vi "Add VI or CTL to lvproj, lvlib, or lvclass.vi"(0 "Add into Project?":bool, 1 "VI Ref":refnum<vi>, 2 "lvlib or lvclass Ref":refnum<vi>, 5 "Add into lvlib or lvclass?":bool, 7 "Add into Virtual Folder?":bool, 9 "Virtual Folder Search Results":T3, 11 "error in":errorcluster, 12 "Initial State":T2, 13 "User VI Owner Status":T1, 14 "Project Name":string) -> (15 "error out":errorcluster)   [LabVIEW 2022 SP3]
doc: "This VI adds or inserts the newly created VI or CTL to a lvproj, lvlib, or lvclass, as per what the user selected. This VI can also insert the newly created VI or CTL into a Virtual Folder, if that's what the user selected.\n\nThis VI handles everything to do with inserting the newly created file into a Project Item.\n\nThis VI assumes that the newly created VI has already been saved to disk (i.e. already exists on disk).\n\nAcronyms\nATP = \"Add To Project?\" checkbox\nATO = \"Add To Owner?\" checkbox (lvlib or lvclass)\nATVF = \"Add To Virtual Folder?\" checkbox"
uses:
  DFS Output (cluster).ctl
  GUI Manager Module/Initial State (enum).ctl
  Owner Status (enum).ctl
  Virtual Folder Type (enum).ctl
panel:
  # "Development\ncontrols/indicators useful for development and testing, but which are not outputs of the VI"
  # "Input\nInputs to the VI"
  # "Output\nOutputs of the VI"
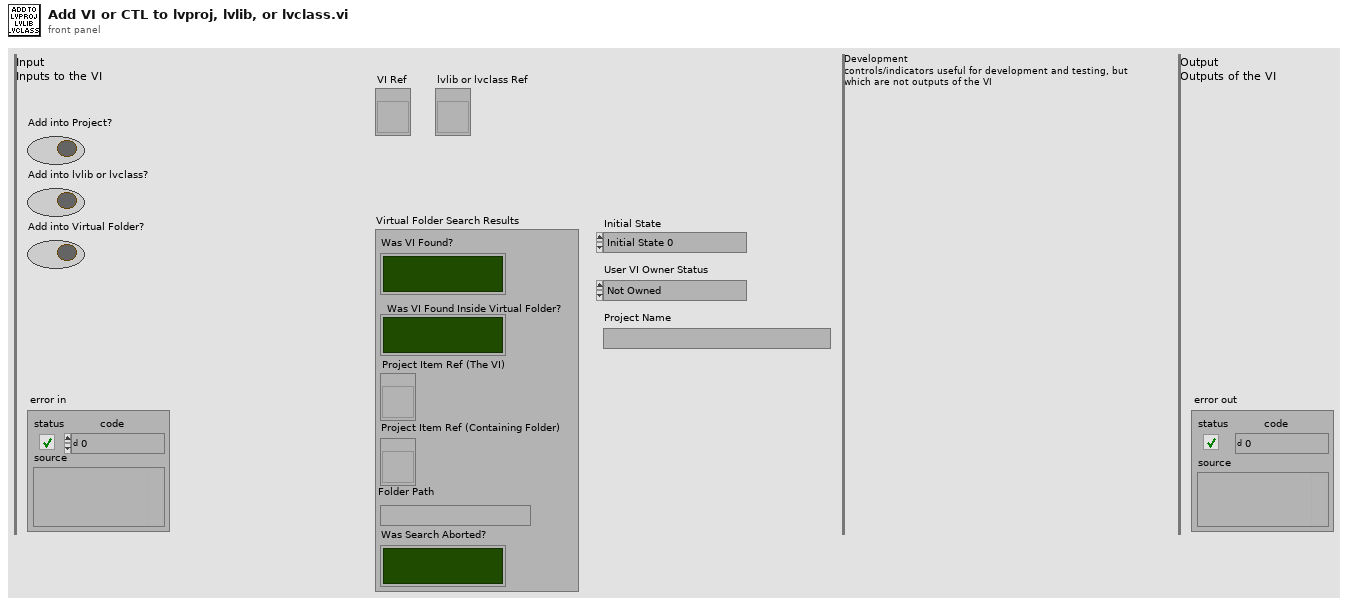
[diagram p1: front panel]
types:
  T1 = typedef "Owner Status (enum).ctl" = enum16{"Not Owned", "Owned by Library (lvlib)", "Owned by Class (lvclass)"}
  T2 = typedef "Initial State (enum).ctl" = enum16{"Initial State 0", "Initial State 1", "Initial State 2", "Initial State 3", "Initial State 4", "Initial State 5", "Initial State 6", "Initial State 7", "Initial State 8", "Initial State 9", "Initial State 10", "Initial State 11", "Initial State 12", "Initial State 13", "Initial State 14", "Initial State 15"}
  T3 = typedef "DFS Output (cluster).ctl" = cluster{"Was VI Found?":bool, "Was VI Found Inside Virtual Folder?":bool, "Project Item Ref (The VI)":refnum<vi>, "Project Item Ref (Containing Folder)":refnum<vi>, "Folder Path":string, "Was Search Aborted?":bool}
  T4 = typedef "Virtual Folder Type (enum).ctl" = enum16{"Owned by lvlib or lvclass", "Owned by lvproj"}
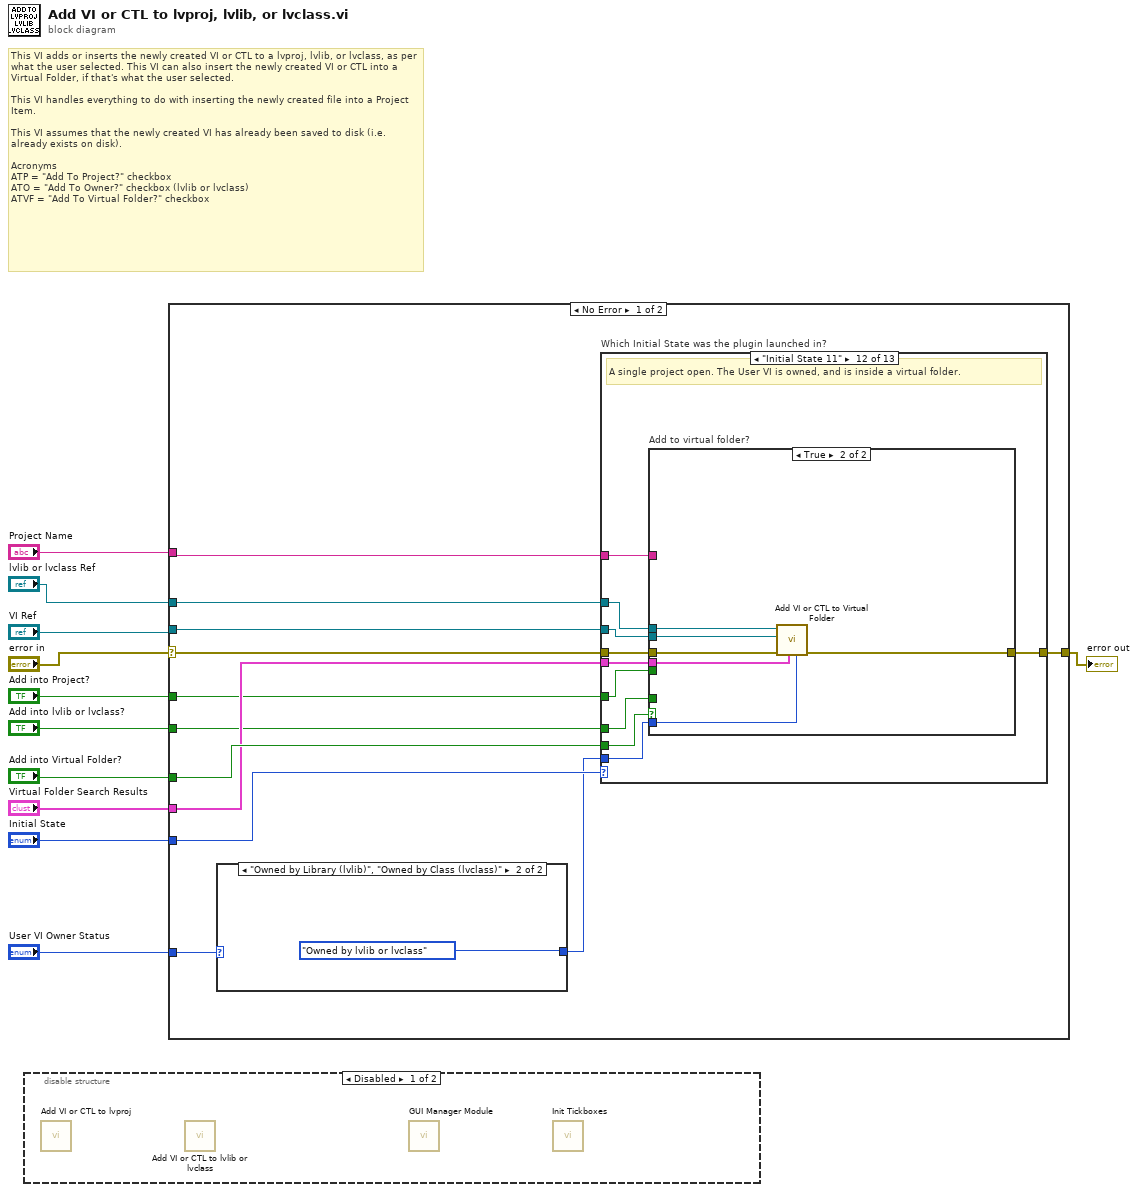
[diagram p0: block diagram]
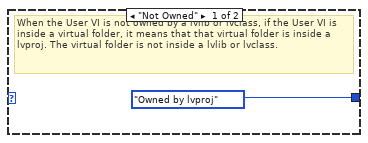
[diagram p2: hidden frame]
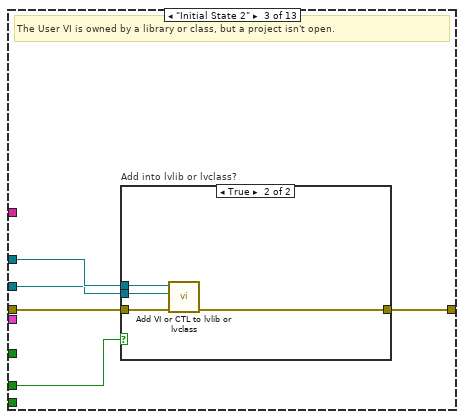
[diagram p5: hidden frame]
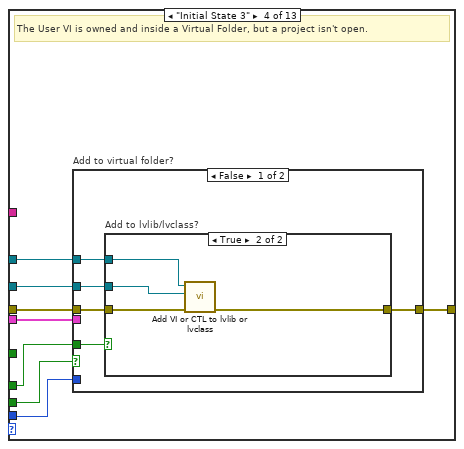
[diagram p7: hidden frame]
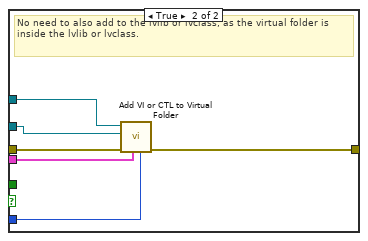
[diagram p9: hidden frame]
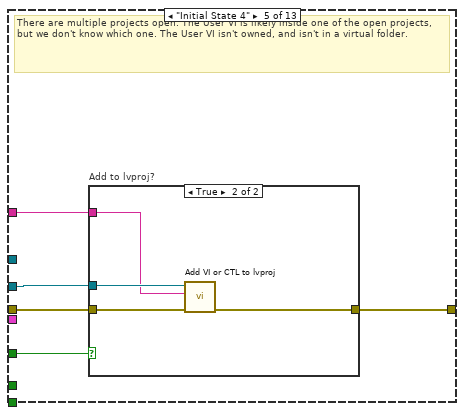
[diagram p10: hidden frame]
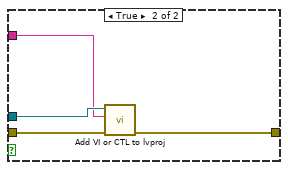
[diagram p14: hidden frame]
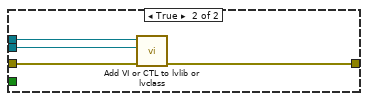
[diagram p15: hidden frame]
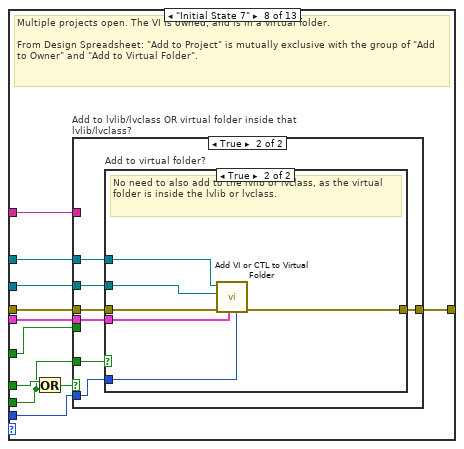
[diagram p16: hidden frame]
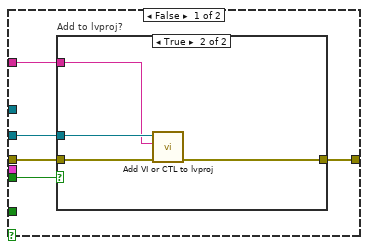
[diagram p17: hidden frame]
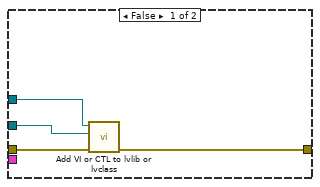
[diagram p19: hidden frame]
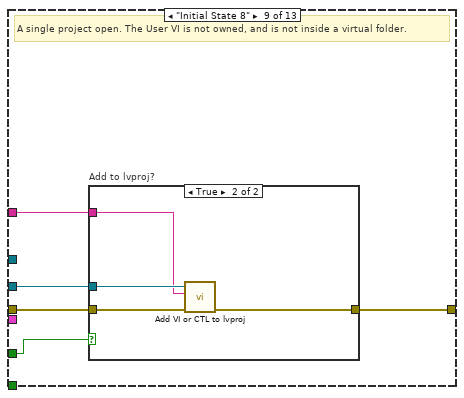
[diagram p20: hidden frame]
diagram:
  # "This VI adds or inserts the newly created VI or CTL to a lvproj, lvlib, or lvclass, as per what the user selected. This VI can also insert the newly created VI or CTL into a Virtual Folder, if that's what the user selected.\n\nThis VI handles everything to do with inserting the newly created file into a Project Item.\n\nThis VI assumes that the newly created VI has already been saved to disk (i.e. already exists on disk).\n\nAcronyms\nATP = \"Add To Project?\" checkbox\nATO = \"Add To Owner?\" checkbox (lvlib or lvclass)\nATVF = \"Add To Virtual Folder?\" checkbox"
  n1 = disable-structure shown="Disabled" {
    frame Disabled {
      n2 = call "Add VI or CTL to lvproj.vi"() -> ()  [unwired: 11 in, 1 out]
      n3 = call "Add VI or CTL to lvlib or lvclass.vi"() -> ()  [unwired: 11 in, 1 out]
      n4 = call "GUI Manager Module.vi"() -> ()  [unwired: 11 in, 1 out]
      n5 = call "Init Tickboxes.vi"() -> ()  [unwired: 11 in, 1 out]
    }
    frame Enabled {
    }
  }
  n6 = case shown="No Error" "error in" {
    selector: "error in" -> [w23 w226]
    tunnel: [w21 w226] -> w10
    tunnel: "lvlib or lvclass Ref" -> [w20 _]
    tunnel: "VI Ref" -> [w19 _]
    tunnel: "Virtual Folder Search Results" -> [w17 _]
    tunnel: "Add into Virtual Folder?" -> [w18 _]
    tunnel: "Initial State" -> [w22 _]
    tunnel: "Add into Project?" -> [w13 _]
    tunnel: "Add into lvlib or lvclass?" -> [w16 _]
    tunnel: "User VI Owner Status" -> [w15 _]
    tunnel: "Project Name" -> [w12 _]
    frame No Error {
      n7 = case shown="\"Owned by Library (lvlib)\", \"Owned by Class (lvclass)\"" w15 {
        tunnel: [Virtual_Folder_Type_(enum)."Owned by lvproj" ("Virtual Folder Type") Virtual_Folder_Type_(enum)."Owned by lvlib or lvclass" ("Virtual Folder Type")] -> w14
        frame "Not Owned" {
          # "When the User VI is not owned by a lvlib or lvclass, if the User VI is inside a virtual folder, it means that that virtual folder is inside a lvproj. The virtual folder is not inside a lvlib or lvclass."
        }
        frame "Owned by Library (lvlib)", "Owned by Class (lvclass)" {
        }
      }
      n8 = case "Which Initial State was the plugin launched in?" shown="\"Initial State 11\"" w22 {
        tunnel: w23 -> [w26 w27 w31 w45 w66 w72 w79 w104 w136 w150 w173 w197 w225]
        tunnel: [w26 w27 w32 w44 w65 w72 w78 w103 w135 w149 w172 w196 w225] -> w21
        tunnel: w20 -> [_ _ w30 w39 _ _ w77 w94 _ w144 w170 w195 _]
        tunnel: w19 -> [_ _ w29 w38 w63 _ w76 w98 w133 w145 w169 w194 _]
        tunnel: w18 -> [_ _ _ w43 _ _ _ w97 _ w148 _ w192 _]
        tunnel: w17 -> [_ _ _ w41 _ _ _ w96 _ w143 _ w191 _]
        tunnel: w16 -> [_ _ w28 w40 _ _ w75 w102 _ _ w171 w188 _]
        tunnel: w14 -> [_ _ _ w42 _ _ _ w95 _ w142 _ w190 _]
        tunnel: w13 -> [_ _ _ _ w64 _ w74 w100 w134 w147 w167 w189 _]
        tunnel: w12 -> [_ _ _ _ w62 _ w73 w99 w132 w146 w168 w193 _]
        frame "Initial State 0" {
          # "Do nothing. The ATP, ATO, and ATVF checkboxes should be disabled."
          # "The User VI is opened on its own. It's not part of a library, class, or project."
        }
        frame "Initial State 1" {
          # "Impossible Initial State. Expected to never occur."
        }
        frame "Initial State 2" {
          # "The User VI is owned by a library or class, but a project isn't open."
          n9 = case "Add into lvlib or lvclass?" shown="True" w28 {
            tunnel: [w33 w37] -> w32
            tunnel: w31 -> [w33 w36]
            tunnel: w30 -> [_ w35]
            tunnel: w29 -> [_ w34]
            frame False {
            }
            frame True {
              n10 = call "Add VI or CTL to lvlib or lvclass.vi"("error in"=w36, "VI Ref"=w34, "lvlib or lvclass Ref"=w35) -> ("error out"=w37:errorcluster)  [unwired: 8 in]
            }
          }
        }
        frame "Initial State 3" {
          # "The User VI is owned and inside a Virtual Folder, but a project isn't open."
          n11 = case "Add to virtual folder?" shown="False" w43 {
            tunnel: w45 -> [w50 w61]
            tunnel: [w49 w60] -> w44
            tunnel: w42 -> [_ w59]
            tunnel: w41 -> [_ w58]
            tunnel: w40 -> [w48 _]
            tunnel: w39 -> [w47 w57]
            tunnel: w38 -> [w46 w56]
            frame False {
              n12 = case "Add to lvlib/lvclass?" shown="True" w48 {
                tunnel: w50 -> [w51 w55]
                tunnel: [w51 w54] -> w49
                tunnel: w47 -> [_ w53]
                tunnel: w46 -> [_ w52]
                frame False {
                  # "The user selected not to insert the newly created VI anywhere."
                }
                frame True {
                  n13 = call "Add VI or CTL to lvlib or lvclass.vi"("error in"=w55, "VI Ref"=w52, "lvlib or lvclass Ref"=w53) -> ("error out"=w54:errorcluster)  [unwired: 8 in]
                }
              }
            }
            frame True {
              # "No need to also add to the lvlib or lvclass, as the virtual folder is inside the lvlib or lvclass."
              n14 = call "Add VI or CTL to Virtual Folder.vi"("Virtual Folder Type"=w59, "Virtual Folder Search Results"=w58, "error in"=w61, "VI Ref"=w56, "lvlib or lvclass Ref"=w57) -> ("error out"=w60:errorcluster)  [unwired: 6 in]
            }
          }
        }
        frame "Initial State 4" {
          # "There are multiple projects open. The User VI is likely inside one of the open projects, but we don't know which one. The User VI isn't owned, and isn't in a virtual folder."
          n15 = case "Add to lvproj?" shown="True" w64 {
            tunnel: w66 -> [w67 w71]
            tunnel: [w67 w70] -> w65
            tunnel: w63 -> [_ w69]
            tunnel: w62 -> [_ w68]
            frame False {
              # "The user selected not to insert the newly created VI anywhere."
            }
            frame True {
              n16 = call "Add VI or CTL to lvproj.vi"("error in"=w71, "Project Name"=w68, "Reference of newly created VI or CTL"=w69) -> ("error out"=w70:errorcluster)  [unwired: 8 in]
            }
          }
        }
        frame "Initial State 5" {
          # "Impossible Initial State. Expected to never occur."
        }
        frame "Initial State 6" {
          # "Multiple projects open. The VI is owned, but isn't in a virtual folder.\n\nFrom Design Spreadsheet: Ticking \"Add to Owner\" and \"Add to Project\" is mutually exclusive (only one checkbox can be ticked at a given time)"
          n17 = case "Add to lvlib/lvclass?" shown="False" w75 {
            tunnel: w79 -> [w84 w93]
            tunnel: [w83 w92] -> w78
            tunnel: w77 -> [_ w91]
            tunnel: w76 -> [w81 w90]
            tunnel: w74 -> [w82 _]
            tunnel: w73 -> [w80 _]
            frame False {
              n18 = case "Add to lvproj?" shown="False" w82 {
                tunnel: w84 -> [w85 w89]
                tunnel: [w85 w88] -> w83
                tunnel: w81 -> [_ w87]
                tunnel: w80 -> [_ w86]
                frame False {
                  # "The user selected not to insert the newly created VI anywhere."
                }
                frame True {
                  n19 = call "Add VI or CTL to lvproj.vi"("error in"=w89, "Project Name"=w86, "Reference of newly created VI or CTL"=w87) -> ("error out"=w88:errorcluster)  [unwired: 8 in]
                }
              }
            }
            frame True {
              n20 = call "Add VI or CTL to lvlib or lvclass.vi"("error in"=w93, "VI Ref"=w90, "lvlib or lvclass Ref"=w91) -> ("error out"=w92:errorcluster)  [unwired: 8 in]
            }
          }
        }
        frame "Initial State 7" {
          # "Multiple projects open. The VI is owned, and is in a virtual folder.\n\nFrom Design Spreadsheet: \"Add to Project\" is mutually exclusive with the group of \"Add to Owner\" and \"Add to Virtual Folder\"."
          n21 = Or(x=w102, y=w97) -> (x .or. y?=w101:bool)
          n22 = case "Add to lvlib/lvclass OR virtual folder inside that lvlib/lvclass?" shown="True" w101 {
            tunnel: [w108 w120] -> w103
            tunnel: w104 -> [w109 w121]
            tunnel: w100 -> [w107 _]
            tunnel: w99 -> [w106 _]
            tunnel: w98 -> [w105 w116]
            tunnel: w97 -> [_ w119]
            tunnel: w96 -> [_ w118]
            tunnel: w95 -> [_ w117]
            tunnel: w94 -> [_ w115]
            frame False {
              n23 = case "Add to lvproj?" shown="True" w107 {
                tunnel: w109 -> [w110 w114]
                tunnel: [w110 w113] -> w108
                tunnel: w105 -> [_ w112]
                tunnel: w106 -> [_ w111]
                frame False {
                  # "The user selected not to insert the newly created VI anywhere."
                }
                frame True {
                  n24 = call "Add VI or CTL to lvproj.vi"("error in"=w114, "Project Name"=w111, "Reference of newly created VI or CTL"=w112) -> ("error out"=w113:errorcluster)  [unwired: 8 in]
                }
              }
            }
            frame True {
              n25 = case "Add to virtual folder?" shown="True" w119 {
                tunnel: w121 -> [w125 w131]
                tunnel: [w124 w130] -> w120
                tunnel: w117 -> [_ w129]
                tunnel: w118 -> [_ w128]
                tunnel: w115 -> [w123 w126]
                tunnel: w116 -> [w122 w127]
                frame False {
                  n26 = call "Add VI or CTL to lvlib or lvclass.vi"("error in"=w125, "VI Ref"=w122, "lvlib or lvclass Ref"=w123) -> ("error out"=w124:errorcluster)  [unwired: 8 in]
                }
                frame True {
                  # "No need to also add to the lvlib or lvclass, as the virtual folder is inside the lvlib or lvclass."
                  n27 = call "Add VI or CTL to Virtual Folder.vi"("Virtual Folder Type"=w129, "Virtual Folder Search Results"=w128, "error in"=w131, "VI Ref"=w127, "lvlib or lvclass Ref"=w126) -> ("error out"=w130:errorcluster)  [unwired: 6 in]
                }
              }
            }
          }
        }
        frame "Initial State 8" {
          # "A single project open. The User VI is not owned, and is not inside a virtual folder."
          n28 = case "Add to lvproj?" shown="True" w134 {
            tunnel: w136 -> [w137 w141]
            tunnel: [w137 w140] -> w135
            tunnel: w133 -> [_ w139]
            tunnel: w132 -> [_ w138]
            frame False {
              # "The user selected not to insert the newly created VI anywhere."
            }
            frame True {
              n29 = call "Add VI or CTL to lvproj.vi"("error in"=w141, "Project Name"=w138, "Reference of newly created VI or CTL"=w139) -> ("error out"=w140:errorcluster)  [unwired: 8 in]
            }
          }
        }
        frame "Initial State 9" {
          # "A single project open. The User VI is not owned, but is inside a virtual folder."
          n30 = case "Add to virtual folder?" shown="False" w148 {
            tunnel: w150 -> [w155 w166]
            tunnel: [w154 w165] -> w149
            tunnel: w144 -> [_ w164]
            tunnel: w145 -> [w152 w163]
            tunnel: w147 -> [w153 _]
            tunnel: w146 -> [w151 _]
            tunnel: w143 -> [_ w162]
            tunnel: w142 -> [_ w161]
            frame False {
              n31 = case "Add to lvproj?" shown="True" w153 {
                tunnel: w155 -> [w156 w160]
                tunnel: [w156 w159] -> w154
                tunnel: w152 -> [_ w158]
                tunnel: w151 -> [_ w157]
                frame False {
                  # "The user selected not to insert the newly created VI anywhere."
                }
                frame True {
                  n32 = call "Add VI or CTL to lvproj.vi"("error in"=w160, "Project Name"=w157, "Reference of newly created VI or CTL"=w158) -> ("error out"=w159:errorcluster)  [unwired: 8 in]
                }
              }
            }
            frame True {
              n33 = call "Add VI or CTL to Virtual Folder.vi"("Virtual Folder Type"=w161, "Virtual Folder Search Results"=w162, "error in"=w166, "VI Ref"=w163, "lvlib or lvclass Ref"=w164) -> ("error out"=w165:errorcluster)  [unwired: 6 in]
            }
          }
        }
        frame "Initial State 10" {
          # "A single project open. The User VI is owned, but is not inside a virtual folder."
          n34 = case "Add to lvlib/lvclass?" shown="False" w171 {
            tunnel: w173 -> [w178 w187]
            tunnel: [w177 w186] -> w172
            tunnel: w170 -> [_ w185]
            tunnel: w169 -> [w175 w184]
            tunnel: w167 -> [w176 _]
            tunnel: w168 -> [w174 _]
            frame False {
              n35 = case "Add to lvproj?" shown="False" w176 {
                tunnel: w178 -> [w179 w183]
                tunnel: [w179 w182] -> w177
                tunnel: w175 -> [_ w181]
                tunnel: w174 -> [_ w180]
                frame False {
                  # "The user selected not to insert the newly created VI anywhere."
                }
                frame True {
                  n36 = call "Add VI or CTL to lvproj.vi"("error in"=w183, "Project Name"=w180, "Reference of newly created VI or CTL"=w181) -> ("error out"=w182:errorcluster)  [unwired: 8 in]
                }
              }
            }
            frame True {
              n37 = call "Add VI or CTL to lvlib or lvclass.vi"("error in"=w187, "VI Ref"=w184, "lvlib or lvclass Ref"=w185) -> ("error out"=w186:errorcluster)  [unwired: 8 in]
            }
          }
        }
        frame "Initial State 11" {
          # "A single project open. The User VI is owned, and is inside a virtual folder."
          n38 = case "Add to virtual folder?" shown="True" w192 {
            tunnel: w197 -> [w204 w224]
            tunnel: [w203 w223] -> w196
            tunnel: w195 -> [w198 w222]
            tunnel: w194 -> [w201 w221]
            tunnel: w189 -> [w202 _]
            tunnel: w193 -> [w200 _]
            tunnel: w191 -> [_ w220]
            tunnel: w190 -> [_ w219]
            tunnel: w188 -> [w199 _]
            frame False {
              n39 = case "Add to lvlib/lvclass?" shown="False" w199 {
                tunnel: w204 -> [w209 w218]
                tunnel: [w208 w217] -> w203
                tunnel: w202 -> [w207 _]
                tunnel: w201 -> [w206 w215]
                tunnel: w200 -> [w205 _]
                tunnel: w198 -> [_ w216]
                frame False {
                  n40 = case "Add to lvproj?" shown="False" w207 {
                    tunnel: w209 -> [w210 w214]
                    tunnel: [w210 w213] -> w208
                    tunnel: w206 -> [_ w212]
                    tunnel: w205 -> [_ w211]
                    frame False {
                      # "The user selected not to insert the newly created VI anywhere."
                    }
                    frame True {
                      n41 = call "Add VI or CTL to lvproj.vi"("error in"=w214, "Project Name"=w211, "Reference of newly created VI or CTL"=w212) -> ("error out"=w213:errorcluster)  [unwired: 8 in]
                    }
                  }
                }
                frame True {
                  n42 = call "Add VI or CTL to lvlib or lvclass.vi"("error in"=w218, "VI Ref"=w215, "lvlib or lvclass Ref"=w216) -> ("error out"=w217:errorcluster)  [unwired: 8 in]
                }
              }
            }
            frame True {
              n43 = call "Add VI or CTL to Virtual Folder.vi"("Virtual Folder Type"=w219, "Virtual Folder Search Results"=w220, "error in"=w224, "VI Ref"=w221, "lvlib or lvclass Ref"=w222) -> ("error out"=w223:errorcluster)  [unwired: 6 in]
            }
          }
        }
        frame "Initial State 12".."Initial State 15" {
          # "Impossible Initial State. Expected to never occur."
        }
      }
    }
    frame Error {
    }
  }
  "error out" <- w10
